vi "Test.vi"() -> ()   [LabVIEW 2023]
uses:
  S7Plc.ctl
  D:/Projects/S7View/S7Lib/bin/Debug/S7Lib.dll
  S7Lib/bin/Debug/S7Lib.dll
panel:
  in  "布尔":bool
  out "S7PLC":T1={"title"="XXX PLC", "id"=0, "ip"="192.168.10.10", "type"=40, "rack"=0, "slot"=0, "isRunning"=FALSE, "isConnected"=FALSE, "msg"="", "label_status"="STOP", "lable_link"="未连接"} {"type" items=["S7200"=0, "Logo0BA8"=1, "S7200Smart"=2, "S7300"=10, "S7400"=20, "S71200"=30, "S71500"=40]}
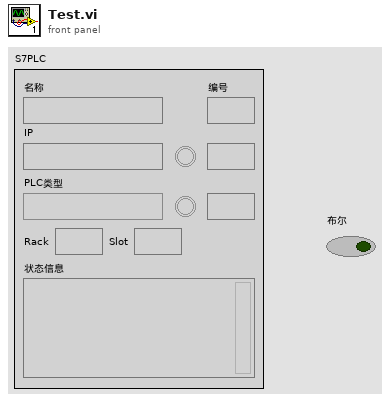
[diagram p1: front panel]
types:
  T1 = typedef "S7Plc.ctl" = cluster{"title":string, "id":i16, "ip":string, "type":i16, "rack":i16, "slot":i16, "isRunning":bool, "isConnected":bool, "msg":string, "label_status":string, "lable_link":string}
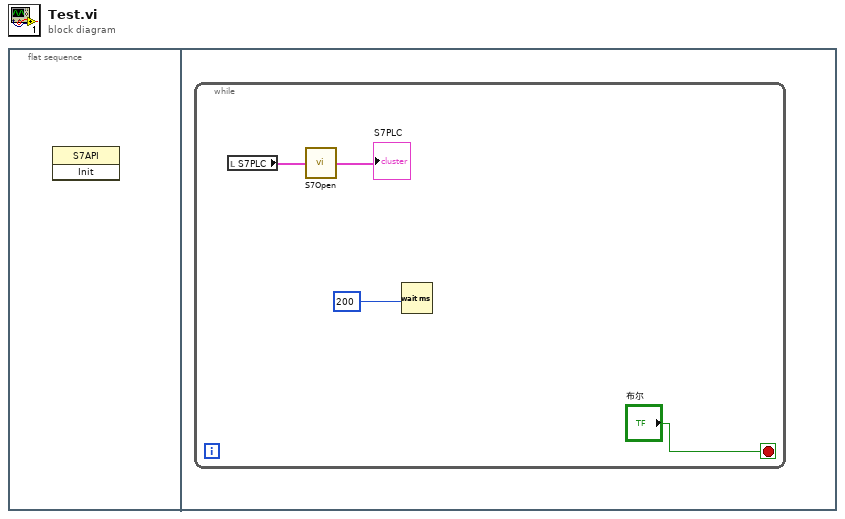
[diagram p0: block diagram]
diagram:
  n1 = flat-sequence {
    frame #0 {
      n2 = invoke on="调用节点" class="S7API" method="Init"() -> ()  [unwired: 3 in, 3 out]
    }
    frame #1 {
      n3 = while {
        stop <- "布尔" stop-if-true
        n4 = local read "S7PLC"() -> (w4:T1)
        n5 = call "S7Open.vi"("Input"=w4) -> ("Output"=→"S7PLC":T1)
        n6 = Wait (ms)(milliseconds to wait=200) -> ()  [unwired: 1 out]
      }
    }
  }
